vi "Get Names.vi"(8 "error in (no error)":errorcluster, 11 "Basic Column Configuration in":refnum<class "Basic Column Configuration.lvclass">) -> (0 "error out":errorcluster, 1 "Column Name":string, 2 "Table Name":string, 3 "Basic Column Configuration out":refnum<class "Basic Column Configuration.lvclass">, 5 "Column Type":T1)   [LabVIEW 2020, in "Basic Columns.lvlib" / "Basic Column Configuration.lvclass"]
uses:
  Basic Column Configuration.lvclass
  Database Interfaces/Database data type.ctl
  Basic Column Configuration.lvclass/Basic Column Configuration.ctl
  Database Interfaces.lvlib
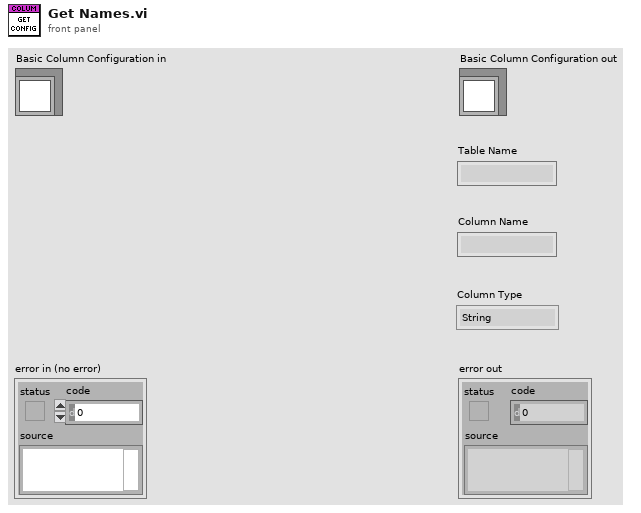
[diagram p1: front panel]
types:
  T1 = typedef "Database Interfaces.lvlib/Database data type.ctl" = enum16{"String", "Long (I32)", "Single (SGL)", "Double (DBL)", "Date/Time", "Binary"}
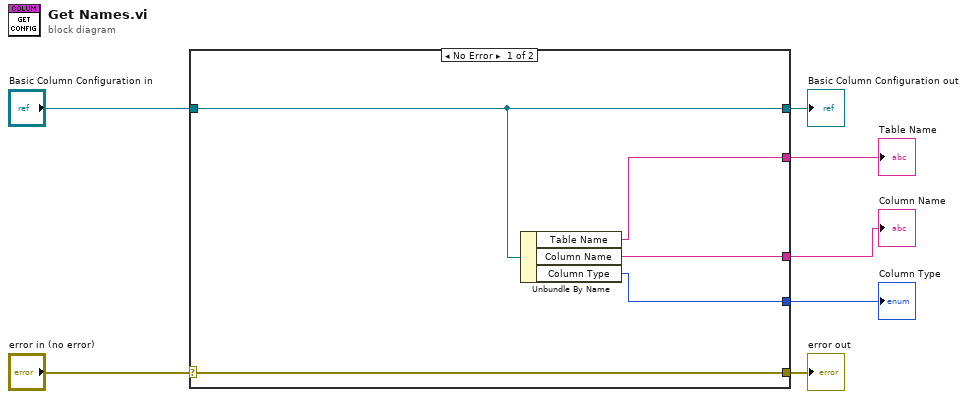
[diagram p0: block diagram]
diagram:
  n1 = case shown="No Error" "error in (no error)" {
    selector: "error in (no error)" -> [w12 w14]
    tunnel: [w12 w14] -> w6
    tunnel: [w11 w13] -> w4
    tunnel: "Basic Column Configuration in" -> [w11 w13]
    tunnel: [w10 _] -> w3
    tunnel: [w9 _] -> w2
    tunnel: [w8 _] -> w1
    frame No Error {
      n2 = Unbundle By Name(w11) -> ("Table Name"=w10:string, "Column Name"=w9:string, "Column Type"=w8:T1)
    }
    frame Error {
    }
  }
  "error out" <- w6
  "Basic Column Configuration out" <- w4
  "Table Name" <- w3
  "Column Name" <- w2
  "Column Type" <- w1
